vi "Configure ALC Search.vi"(0 "VISA resource name":refnum<visa-resource-name>, 1 "Enable Power Protection (F:Disable)":bool, 2 "Power Search Reference (0: Modulated)":u16(ring) items=["Modulated", "Fixed"], 5 "Power Search Mode (0: On)":u16(ring) items=["On", "Off", "Once", "Span"], 7 "Enable Span Power Search (T:Enable)":bool=TRUE, 9 "Span Type (0: Full)":u16(ring) items=["Full", "User"], 11 "error in (no error)":errorcluster, 12 "Span Start Frequency (1 MHz)":dbl=1000000.0, 13 "Span Stop Frequency (2 MHz)":dbl=2000000.0) -> (4 "VISA resource name out":refnum<visa-resource-name>, 15 "error out":errorcluster)   [LabVIEW 2012, in "Agilent PSG MXG Series.lvlib"]
doc: "Configures the internal power search and the span mode.\n\n<B>Notes:</B>\n(1) This VI is valid only when ALC is OFF."
uses:
  <instrlib>/Agilent PSG MXG Series/Agilent PSG MXG Series.lvlib
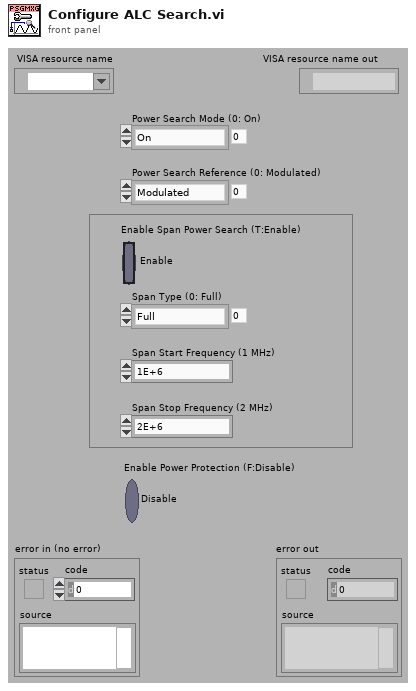
[diagram p1: front panel]
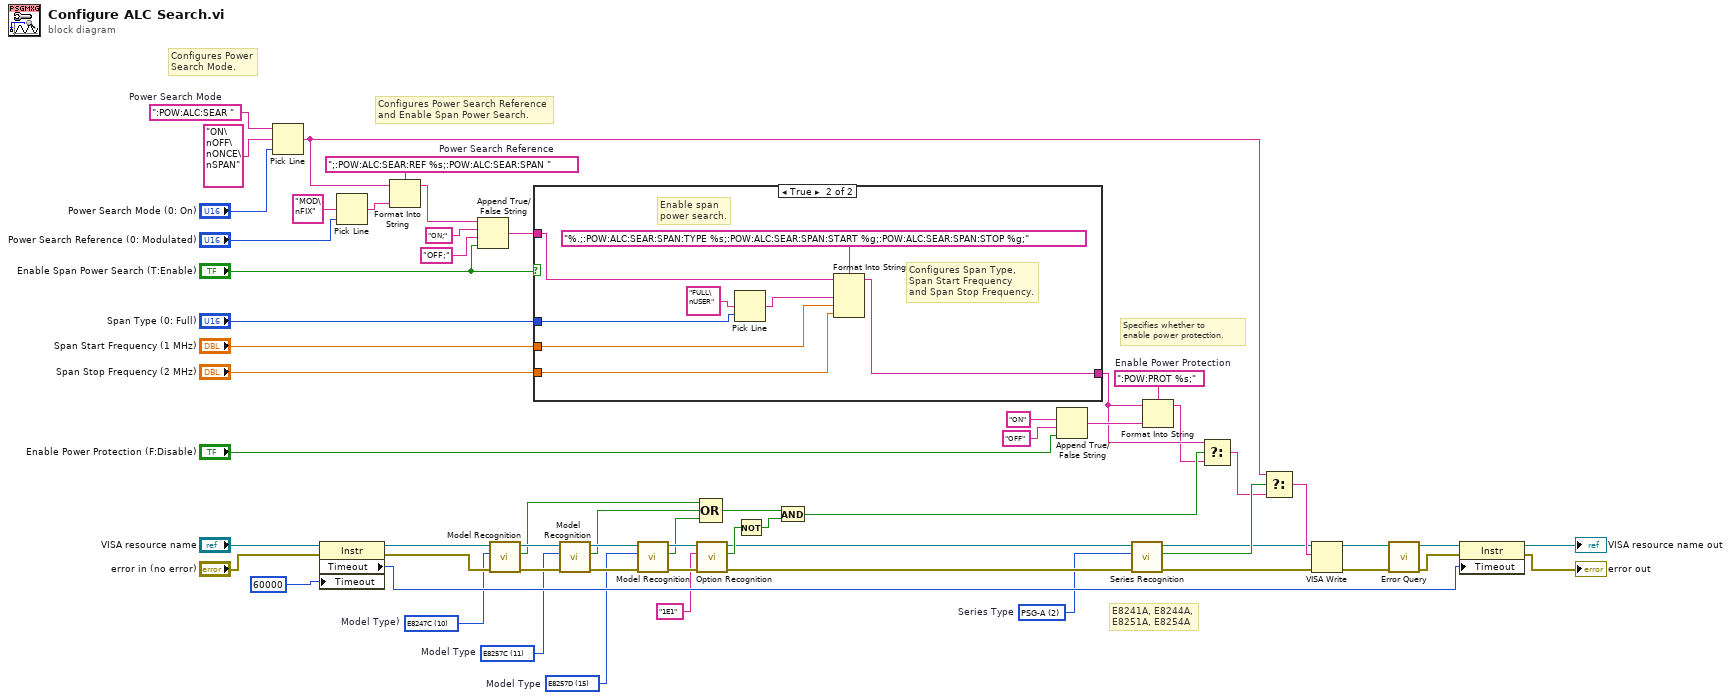
[diagram p0: block diagram]
diagram:
  w1 = u16 2 items=["MXG-A", "PSG", "PSG-A", "PSG-C", "PSG-D", "MXG-B", "EXG"]  # Series Type
  w2 = u16 15 items=["N5181A"=0, "N5182A"=1, "N5183A"=2, "N5161A"=3, "N5162A"=4, "E8241A"=5, "E8244A"=6, "E8251A"=7, "E8254A"=8, "E8247C"=10, "E8257C"=11, "E8267C"=12, "E8257D"=15, "E8267D"=16, "N5171B"=17, "N5172B"=18, "N5181B"=19, "N5182B"=20]  # Model Type
  w3 = u16 11 items=["N5181A"=0, "N5182A"=1, "N5183A"=2, "N5161A"=3, "N5162A"=4, "E8241A"=5, "E8244A"=6, "E8251A"=7, "E8254A"=8, "E8247C"=10, "E8257C"=11, "E8267C"=12, "E8257D"=15, "E8267D"=16, "N5171B"=17, "N5172B"=18, "N5181B"=19, "N5182B"=20]  # Model Type
  w4 = u16 10 items=["N5181A"=0, "N5182A"=1, "N5183A"=2, "N5161A"=3, "N5162A"=4, "E8241A"=5, "E8244A"=6, "E8251A"=7, "E8254A"=8, "E8247C"=10, "E8257C"=11, "E8267C"=12, "E8257D"=15, "E8267D"=16, "N5171B"=17, "N5172B"=18, "N5181B"=19, "N5182B"=20]  # Model Type)
  w45 = ":POW:PROT %s;"  # Enable Power Protection
  w57 = ";:POW:ALC:SEAR:REF %s;:POW:ALC:SEAR:SPAN "  # Power Search Reference
  w60 = ":POW:ALC:SEAR "  # Power Search Mode
  # "E8241A, E8244A,\nE8251A, E8254A"
  # "Specifies whether to\nenable power protection."
  # "Configures Power Search Reference\nand Enable Span Power Search."
  # "Configures Power\nSearch Mode."
  n1 = Pick Line(string ("")=w60, multi-line string="ON\nOFF\nONCE\nSPAN", line index="Power Search Mode (0: On)") -> (output string=w36:string)
  n2 = property class="Instr"(reference="VISA resource name", error in="error in (no error)", "Timeout"=u32 60000 ("General Settings:Timeout Value")) -> (reference out=w25:refnum<visa-resource-name>, error out=w24:errorcluster, "Timeout"=w28:u32)
  n3 = Pick Line(multi-line string="MOD\nFIX", line index="Power Search Reference (0: Modulated)") -> (output string=w56:string)  [unwired: 1 out]
  n4 = Format Into String(format string=w57, initial string=w36, w56) -> (resulting string=w53:string)  [unwired: 1 in, 1 out]
  n5 = Append True/False String(1:"Enable Span Power Search (T:Enable)", 2:"OFF;" ("false string"), 3:"ON;" ("true string"), 4:w53) -> (0:w49:string)
  n6 = call <instrlib>:"Model Recognition.vi"("error in (no error)"=w24, "Model Type (0: N5181A)"=w4, "VISA resource name"=w25) -> ("error out"=w22:errorcluster, "Is Model Correct"=w16:bool, "VISA resource name out"=w23:refnum<visa-resource-name>)  [unwired: 6 out]
  n7 = case shown="True" "Enable Span Power Search (T:Enable)" {
    tunnel: w49 -> [w61 w69]
    tunnel: "Span Type (0: Full)" -> [_ w65]
    tunnel: "Span Start Frequency (1 MHz)" -> [_ w64]
    tunnel: "Span Stop Frequency (2 MHz)" -> [_ w63]
    tunnel: [w61 w62] -> w8
    frame False {
      # "Disable span power search."
    }
    frame True {
      # "Configures Span Type,\nSpan Start Frequency\nand Span Stop Frequency."
      # "Enable span\npower search."
      n8 = Pick Line(multi-line string="FULL\nUSER", line index=w65) -> (output string=w67:string)  [unwired: 1 out]
      n9 = Format Into String(format string="%.;:POW:ALC:SEAR:SPAN:TYPE %s;:POW:ALC:SEAR:SPAN:START %g;:POW:ALC:SEAR:SPAN:STOP %g;", initial string=w69, w67, w64, w63) -> (resulting string=w62:string)  [unwired: 1 in, 1 out]
    }
  }
  n10 = call <instrlib>:"Model Recognition.vi"("error in (no error)"=w22, "Model Type (0: N5181A)"=w3, "VISA resource name"=w23) -> ("error out"=w20:errorcluster, "Is Model Correct"=w15:bool, "VISA resource name out"=w21:refnum<visa-resource-name>)  [unwired: 6 out]
  n11 = call <instrlib>:"Model Recognition.vi"("error in (no error)"=w20, "Model Type (0: N5181A)"=w2, "VISA resource name"=w21) -> ("error out"=w18:errorcluster, "Is Model Correct"=w14:bool, "VISA resource name out"=w19:refnum<visa-resource-name>)  [unwired: 6 out]
  n12 = call <instrlib>:"Option Recognition.vi"("error in (no error)"=w18, "Option (\"\")"="1E1" ("Option (\"\")"), "VISA resource name"=w19) -> ("error out"=w5:errorcluster, "Is Option Installed"=w13:bool, "VISA resource name out"=w6:refnum<visa-resource-name>)  [unwired: 6 out]
  n13 = Compound Arithmetic op=OR(w16, w15, w14) -> (w12:bool)
  n14 = Not(x=w13) -> (.not. x?=w11:bool)
  n15 = And(x=w12, y=w11) -> (x .and. y?=w9:bool)
  n16 = Append True/False String(1:"Enable Power Protection (F:Disable)", 2:"OFF" ("false string"), 3:"ON" ("true string")) -> (0:w44:string)  [unwired: 1 out]
  n17 = call <instrlib>:"Series Recognition.vi"("error in (no error)"=w5, "Series Type (0: MXG)"=w1, "VISA resource name"=w6) -> ("error out"=w37:errorcluster, "Is Series Correct"=w39:bool, "VISA resource name out"=w38:refnum<visa-resource-name>)  [unwired: 1 in, 5 out]
  n18 = Format Into String(format string=w45, initial string=w8, w44) -> (resulting string=w7:string)  [unwired: 1 in, 1 out]
  n19 = Select(t=w8, s=w9, f=w7) -> (s? t:f=w10:string)
  n20 = Select(t=w36, s=w39, f=w10) -> (s? t:f=w40:string)
  n21 = VISA Write(VISA resource name=w38, write buffer=w40, error in (no error)=w37) -> (VISA resource name out=w35:refnum<visa-resource-name>, error out=w34:errorcluster)  [unwired: 1 out]
  n22 = call <instrlib>:"Error Query.vi"("error in (no error)"=w34, "VISA resource name"=w35) -> ("error out"=w29:errorcluster, "VISA resource name out"=w30:refnum<visa-resource-name>)  [unwired: 8 out]
  n23 = property class="Instr"(reference=w30, error in=w29, "Timeout"=w28) -> (reference out=→"VISA resource name out":refnum<visa-resource-name>, error out=→"error out":errorcluster)
